vi "FilterWheelSubVi.vi"(1 "Position set":i32=5, 2 "Serial Port":string) -> (0 "Position get":i32)   [LabVIEW 2018]
doc: "This example shows how to acquire a power measurement using the VIs of the driver."
uses:
  Thorlabs_FW102C/Thorlabs_FW102C.lvlib
panel:
  out "COM Ports":string[](array[string])
  # "(c) 2015 <Thorlabs>.  ALL RIGHTS RESERVED."
  # "Connect"
  # "Set data"
  # "Read data"
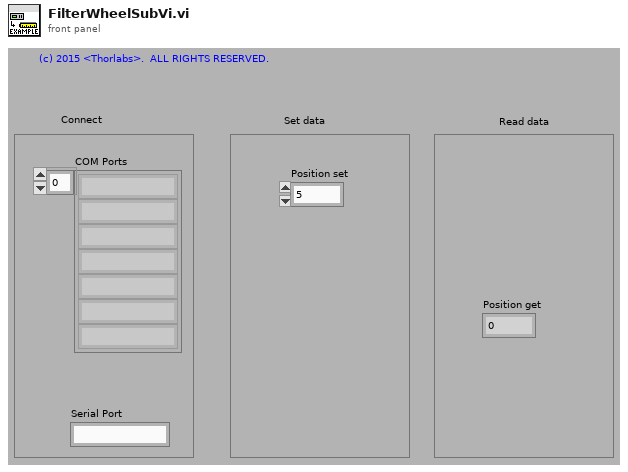
[diagram p1: front panel]
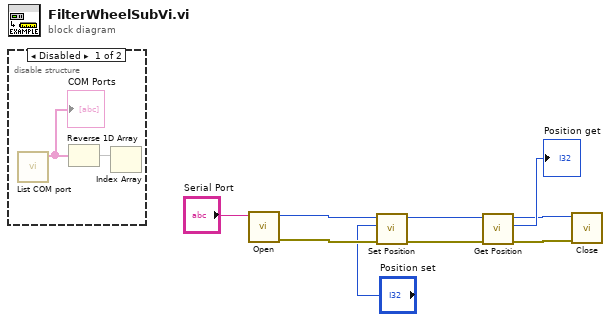
[diagram p0: block diagram]
diagram:
  n1 = disable-structure shown="Disabled" {
    frame Disabled {
      n2 = call "List COM port.vi"() -> ("COM Ports"=w11:string[])  [unwired: 10 in, 1 out]
      "COM Ports" <- w11
      n3 = Reverse 1D Array(array=w11) -> (reversed array=w10:string[])
      n4 = Index Array(array=w10) -> ()  [unwired: 1 in, 1 out]
    }
    frame Enabled {
    }
  }
  n5 = call "Open.vi"("Serial Port"="Serial Port") -> ("error out"=w8:errorcluster, "FW102C out"=w9:i32)  [unwired: 8 in, 1 out]
  n6 = call "Set Position.vi"("error in (no error)"=w8, "Position"="Position set", "FW102C in"=w9) -> ("error out"=w6:errorcluster, "FW102C out"=w7:i32)  [unwired: 7 in]
  n7 = call "Get Position.vi"("error in (no error)"=w6, "FW102C in"=w7) -> ("error out"=w5:errorcluster, "Position"=→"Position get":i32, "FW102C out"=w3:i32)  [unwired: 7 in]
  n8 = call "Close.vi"("error in (no error)"=w5, "FW102C in"=w3) -> ()  [unwired: 9 in, 1 out]
